vi "Alt_Alpha_Ver 1.0.vi"() -> ()   [LabVIEW 2015]
uses:
  <instrlib>/Keithley 622x LV 2009/Configure/Units/Typedefs/KE622x -- Voltage Meas Units.ctl
  <instrlib>/Keithley 622x LV 2009/Configure/2182 -A/Low Level/Typedefs/KE2182 -- Voltage Ranges.ctl
  <instrlib>/Keithley 622x LV 2009/Configure/2182 -A/Low Level/Typedefs/KE2182 -- Filter Type.ctl
  <instrlib>/Keithley 622x LV 2009/Configure/2182 -A/Low Level/Typedefs/KE2182 -- Filter Count.ctl
  <instrlib>/Keithley 622x LV 2009/Configure/2182 -A/Low Level/Typedefs/KE2182 -- Filter Window.ctl
  <instrlib>/Keithley 622x LV 2009/Configure/2182 -A/Low Level/Typedefs/KE2182 -- NPLCs.ctl
  <instrlib>/Keithley 622x LV 2009/Configure/Units/Typedefs/KE6221 -- PDelta Power Meas Type.ctl
  <instrlib>/Keithley 622x LV 2009/Configure/Delta PDelta DCon Modes/Typedefs/KE6221 -- PDelta Mode Params.ctl
  <instrlib>/Keithley 622x LV 2009/Configure/Delta PDelta DCon Modes/Low Level/Typedefs/KE622x -- Delta PDelta Mode High Level.ctl
  <instrlib>/Keithley 622x LV 2009/Configure/Delta PDelta DCon Modes/Low Level/Typedefs/KE622x -- Delta PDelta Mode Low Level.ctl
  <instrlib>/Keithley 622x LV 2009/Configure/Delta PDelta DCon Modes/Low Level/Typedefs/KE6221 -- PDelta Mode Pulse Width.ctl
  <instrlib>/Keithley 622x LV 2009/Configure/Delta PDelta DCon Modes/Low Level/Typedefs/KE6221 -- PDelta Mode Source Delay.ctl
  <instrlib>/Keithley 622x LV 2009/Configure/Delta PDelta DCon Modes/Low Level/Typedefs/KE622x -- Delta PDelta Mode Num Cycles Mode.ctl
  <instrlib>/Keithley 622x LV 2009/Configure/Delta PDelta DCon Modes/Low Level/Typedefs/KE622x -- Delta PDelta Mode Num Cycles.ctl
  <instrlib>/Keithley 622x LV 2009/Configure/Delta PDelta DCon Modes/Low Level/Typedefs/KE6221 -- PDelta Mode Ranging Mode.ctl
  <instrlib>/Keithley 622x LV 2009/Configure/Delta PDelta DCon Modes/Low Level/Typedefs/KE6221 -- PDelta Mode Num Low Meas.ctl
  <instrlib>/Keithley 622x LV 2009/Configure/Delta PDelta DCon Modes/Low Level/Typedefs/KE6221 -- PDelta Mode Pulse Period.ctl
  <instrlib>/Keithley 622x LV 2009/Utility/Typedefs/KE622x -- Instrument Type.ctl
  <instrlib>/Keithley 622x LV 2009/Keithley 622x.lvlib
panel:
  in  "Power Meas Type":T1
  in  "2812 -A Params In":T7={"Auto Range?"=FALSE, "Man / Selected\nRange"=enum."10mV", "Enable Digital\nFilter?"=FALSE, "Filter Type"=enum."Moving", "Filter Count"=10, "Filter\nWindow (%)"=0.01, "Enable Analog\nFilter?"=FALSE, "NPLCs"=5} {"Filter\nWindow (%)" min=0.0 max=10.0 step=0.01 format="%.2f"; "Filter Count" min=1 max=100; "NPLCs" min=1 max=10}
  in  "Measurement Units":T8
  in  "Measurements control":enum32{"PULSE", " DELTA"}(tab)
  in  "Pulsed Delta Mode Params In":T9={"High Level (A)"=0.001, "Low Level (A)"=0.0, "Pulse Width (s)"=0.00011, "Source Delay (s)"=1.6e-05, "Num Cycles Mode"=enum."Finite Count", "Finite Count"=1, "Ranging Mode"=enum."Best", "Num Low Meas Per Cycle"=enum."1", "Pulse Period (Num PLCs)"=5, "Pulse Sweep Mode Enabled?"=FALSE} {"Pulse Period (Num PLCs)" min=5 max=999990; "Source Delay (s)" min=1.6e-05 max=0.011966 format="%.3p"; "Pulse Width (s)" min=5e-05 max=0.012 format="%.3p"; "Finite Count" min=2 max=65536; "Low Level (A)" min=-0.105 max=0.0 format="%.3p"; "High Level (A)" min=0.0 max=0.105 format="%.3p"}
  in  "Comments":string
  in  "Folder \nPrename":string
  # "Keithley  6221 & 2182A Measurement System"
  # "FILE CONFIGURATION"
  # "PRE EXPERIMENT CONFIGS"
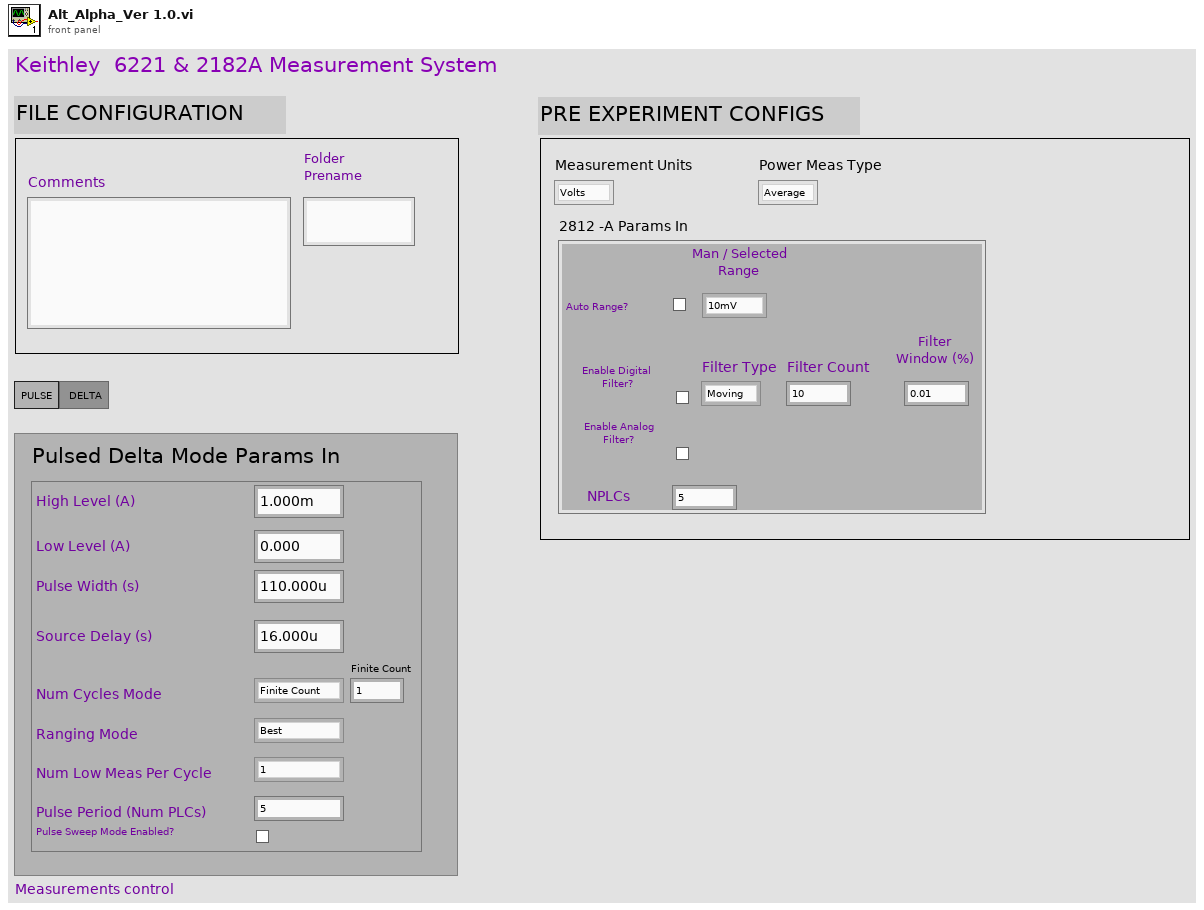
[diagram p1: front panel]
types:
  T1 = typedef "Keithley 622x.lvlib/KE6221 -- PDelta Power Meas Type.ctl" = enum16{"Average", "Peak"}
  T2 = typedef "Keithley 622x.lvlib/KE2182 -- Voltage Ranges.ctl" = enum16{"10mV", "100mV", "1V", "10V", "100V"}
  T3 = typedef "Keithley 622x.lvlib/KE2182 -- Filter Type.ctl" = enum16{"Moving", "Repeat"}
  T4 = typedef "Keithley 622x.lvlib/KE2182 -- Filter Count.ctl" = u32
  T5 = typedef "Keithley 622x.lvlib/KE2182 -- Filter Window.ctl" = dbl
  T6 = typedef "Keithley 622x.lvlib/KE2182 -- NPLCs.ctl" = u32
  T7 = cluster{"Auto Range?":bool, "Man / Selected\nRange":T2, "Enable Digital\nFilter?":bool, "Filter Type":T3, "Filter Count":T4, "Filter\nWindow (%)":T5, "Enable Analog\nFilter?":bool, "NPLCs":T6}
  T8 = typedef "Keithley 622x.lvlib/KE622x -- Voltage Meas Units.ctl" = enum16{"Volts", "Ohms", "Watts", "Siemens"}
  T9 = typedef "Keithley 622x.lvlib/KE6221 -- PDelta Mode Params.ctl" = cluster{"High Level (A)":T10, "Low Level (A)":T11, "Pulse Width (s)":T12, "Source Delay (s)":T13, "Num Cycles Mode":T14, "Finite Count":T15, "Ranging Mode":T16, "Num Low Meas Per Cycle":T17, "Pulse Period (Num PLCs)":T18, "Pulse Sweep Mode Enabled?":bool}
  T10 = typedef "Keithley 622x.lvlib/KE622x -- Delta PDelta Mode High Level.ctl" = dbl
  T11 = typedef "Keithley 622x.lvlib/KE622x -- Delta PDelta Mode Low Level.ctl" = dbl
  T12 = typedef "Keithley 622x.lvlib/KE6221 -- PDelta Mode Pulse Width.ctl" = dbl
  T13 = typedef "Keithley 622x.lvlib/KE6221 -- PDelta Mode Source Delay.ctl" = dbl
  T14 = typedef "Keithley 622x.lvlib/KE622x -- Delta PDelta Mode Num Cycles Mode.ctl" = enum16{"Finite Count", "Infinite"}
  T15 = typedef "Keithley 622x.lvlib/KE622x -- Delta PDelta Mode Num Cycles.ctl" = u32
  T16 = typedef "Keithley 622x.lvlib/KE6221 -- PDelta Mode Ranging Mode.ctl" = enum16{"Best", "Fixed"}
  T17 = typedef "Keithley 622x.lvlib/KE6221 -- PDelta Mode Num Low Meas.ctl" = enum16{"1", "2"}
  T18 = typedef "Keithley 622x.lvlib/KE6221 -- PDelta Mode Pulse Period.ctl" = u32
  T19 = typedef "Keithley 622x.lvlib/KE622x -- Instrument Type.ctl" = enum16{"KE6220", "KE6221"}
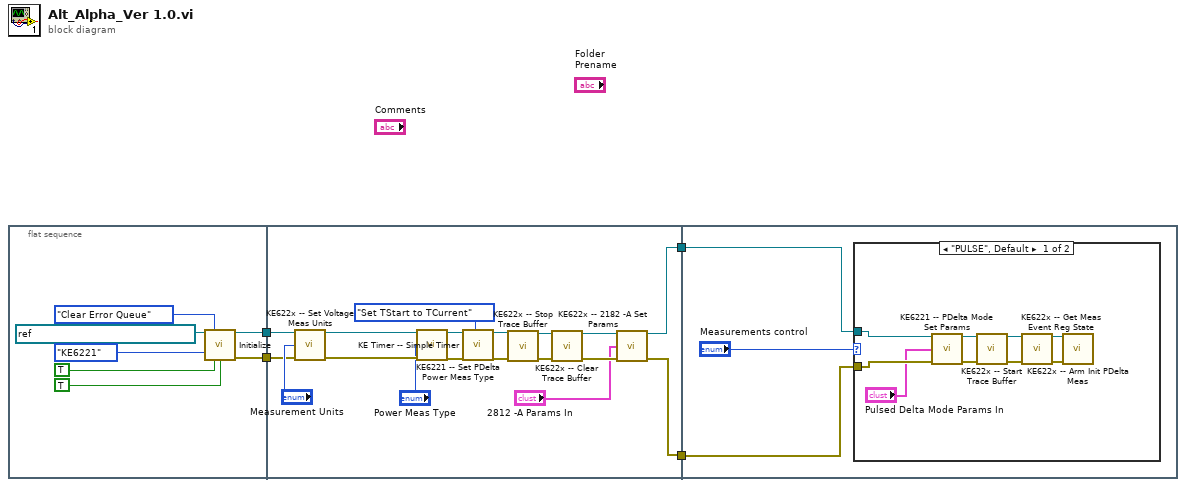
[diagram p0: block diagram]
diagram:
  n1 = flat-sequence {
    tunnel: [w6] -> w4
    tunnel: [w5] -> w3
    tunnel: w4 -> [w28]
    tunnel: w3 -> [w27]
    tunnel: [w18] -> w2
    tunnel: [w17] -> w1
    tunnel: w2 -> [w30]
    tunnel: w1 -> [w31]
    frame #0 {
      n2 = call <instrlib>:"Initialize.vi"("VISA resource name"=refnum<visa-resource-name> "DC_AC_Current_Source_6221", "Error Queue Option"=enum16{"Clear Error Queue", "Error Query"}."Clear Error Queue", "Instrument Type"=KE622x_--_Instrument_Type."KE6221", "ID Query? (T)"=TRUE, "Reset? (T)"=TRUE) -> ("VISA resource name out"=w6:refnum<visa-resource-name>, "error out"=w5:errorcluster)  [unwired: 9 in]
    }
    frame #1 {
      n3 = call <instrlib>:"KE622x -- Set Voltage Meas Units.vi"("Resource In"=w28, "Voltage Meas Units"="Measurement Units", "error in (no error)"=w27) -> ("Resource Out (dupl)"=w16:refnum<visa-resource-name>, "error out"=w15:errorcluster)  [unwired: 11 in]
      n4 = call <instrlib>:"KE6221 -- Set PDelta Power Meas Type.vi"("6221 Resource In"=w16, "Power Meas Type"="Power Meas Type", "error in (no error)"=w15) -> ("6221 Resource Out (dupl)"=w13:refnum<visa-resource-name>, "error out"=w12:errorcluster)  [unwired: 11 in]
      n5 = call <instrlib>:"KE Timer -- Simple Timer.vi"("Resource In"=w13, "error in (no error)"=w12, "Action"=enum16{"Set TStart to TCurrent", "Get Deltas"}."Set TStart to TCurrent") -> ("Resource Out (dupl)"=w25:refnum<visa-resource-name>, "error out (dupl)"=w24:errorcluster)  [unwired: 7 in, 8 out]
      n6 = call <instrlib>:"KE622x -- Stop Trace Buffer.vi"("Resource In"=w25, "error in (no error)"=w24) -> ("Resource Out (dupl)"=w23:refnum<visa-resource-name>, "error out"=w22:errorcluster)  [unwired: 12 in]
      n7 = call <instrlib>:"KE622x -- Clear Trace Buffer.vi"("Resource In"=w23, "error in (no error)"=w22) -> ("Resource Out (dupl)"=w21:refnum<visa-resource-name>, "error out"=w20:errorcluster)  [unwired: 12 in]
      n8 = call <instrlib>:"KE622x -- 2182 -A Set Params.vi"("622x Resource In"=w21, "2812 -A Params In"="2812 -A Params In", "error in (no error)"=w20) -> ("622x Resource Out (dupl)"=w18:refnum<visa-resource-name>, "error out"=w17:errorcluster)  [unwired: 10 in, 1 out]
    }
    frame #2 {
      n9 = case shown="\"PULSE\", Default" "Measurements control" {
        tunnel: w31 -> [w40 _]
        tunnel: w30 -> [w41 _]
        frame "PULSE", Default {
          n10 = call <instrlib>:"KE6221 -- PDelta Mode Set Params.vi"("6221 Resource In"=w41, "Pulsed Delta Mode Params In"="Pulsed Delta Mode Params In", "error in (no error)"=w40) -> ("6221 Resource Out (dupl)"=w38:refnum<visa-resource-name>, "error out"=w37:errorcluster)  [unwired: 10 in, 1 out]
          n11 = call <instrlib>:"KE622x -- Start Trace Buffer.vi"("Resource In"=w38, "error in (no error)"=w37) -> ("Resource Out (dupl)"=w36:refnum<visa-resource-name>, "error out"=w35:errorcluster)  [unwired: 12 in]
          n12 = call <instrlib>:"KE622x -- Get Meas Event Reg State.vi"("VISA Resource In"=w36, "error in (no error)"=w35) -> ("VISA Resource Out (dupl)"=w34:refnum<visa-resource-name>, "error out"=w33:errorcluster)  [unwired: 11 in, 1 out]
          n13 = call <instrlib>:"KE622x -- Arm Init PDelta Meas.vi"("Resource In"=w34, "error in (no error)"=w33) -> ()  [unwired: 12 in, 2 out]
        }
        frame " DELTA" {
        }
      }
    }
  }
